vi "TDMS Find Max Run.vi"(8 "error in (no error)":errorcluster, 11 "TDMS File Path":path) -> (0 "error out":errorcluster, 1 "Found?":bool, 2 "Run ID":string, 3 "TDMS File Path Out":path)   [LabVIEW 2011]
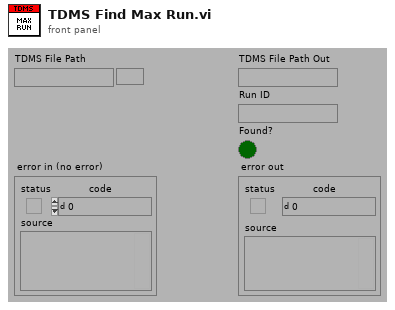
[diagram p1: front panel]
types:
  T1 = enum16{"open", "open or create", "create or replace", "create", "open (read-only)"}
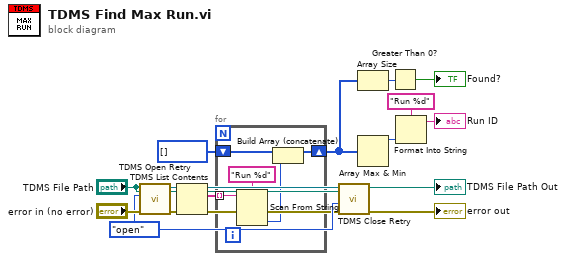
[diagram p0: block diagram]
diagram:
  w15 = T1."open" ("operation (0:open)")
  n1 = call "TDMS Open Retry.vi"("error in (no error)"="error in (no error)", "Operation (0:open)"=w15, "Path"="TDMS File Path") -> ("error out"=w14:errorcluster, "TDMS File Ref"=w13:refnum<k34>)  [unwired: 1 in, 6 out]
  n2 = TDMS List Contents(4:w14, 7:w13) -> (0:w2:errorcluster, 2:w12:string[], 3:w1:refnum<k34>)  [unwired: 1 in, 1 out]
  n3 = for {
    tunnel: w12 -> [w18] mode=indexing
    shift-right: [w21] -> w7
    shift-left: i32[] [] -> [w22]
    n4 = Scan From String(format string="Run %d", input string=w18) -> (output 1=w19:i32)  [unwired: 3 in, 3 out]
    n5 = Build Array (concatenate)(w22, w19) -> (w21:i32[])
  }
  n6 = call "TDMS Close Retry.vi"("TDMS Path"="TDMS File Path", "error in (no error)"=w2, "Operation (0:open)"=w15, "TDMS File Ref"=w1) -> ("error out"=→"error out":errorcluster, "TDMS Path Out"=→"TDMS File Path Out":path)  [unwired: 1 in, 5 out]
  n7 = Array Size(array=w7) -> (size(s)=w6:i32)
  n8 = Array Max & Min(array=w7) -> (max value=w9:i32)  [unwired: 3 out]
  n9 = Greater Than 0?(x=w6) -> (x > 0?=→"Found?":bool)
  n10 = Format Into String(format string="Run %d", w9) -> (resulting string=→"Run ID":string)  [unwired: 2 in, 1 out]
